vi "ds is monitor present.vi"(10 "output_flag":u32, 11 "device_handle":u32) -> (1 "function return":i32, 2 "output_flag out":u32, 3 "device_handle out":u32)   [LabVIEW 2019, in "apdm.lvlib"]
doc: "APDM_EXPORT int apdm_ds_is_monitor_present(apdm_device_handle_t device_handle, uint32_t *output_flag);"
uses:
  apdm.lvlib
  Lee Lab/CP FES Walking 2018/Code/Working/LabVIEW/apdm.dll
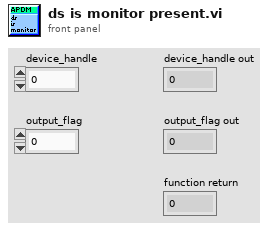
[diagram p1: front panel]
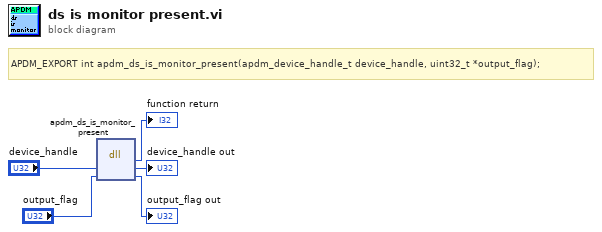
[diagram p0: block diagram]
diagram:
  # "APDM_EXPORT int apdm_ds_is_monitor_present(apdm_device_handle_t device_handle, uint32_t *output_flag);"
  n1 = dll-call lib="C:/Users/jfalesi/Dropbox/Lee Lab/CP FES Walking 2018/Code/Working/LabVIEW/apdm.*" fn="apdm_ds_is_monitor_present"("device_handle"="device_handle", "output_flag"="output_flag") -> (→"function return":i32, "device_handle"=→"device_handle out":u32, "output_flag"=→"output_flag out":u32)  [unwired: 3 in, 2 out]
